vi "BCD to DEC.vi"(11 "BCD":u8) -> (3 "DEC":u16)   [LabVIEW 2014, in "LMH-Toolbox.lvlib"]
doc: "Convert a binary coded decimal to a decimal number."
uses:
  <vilib>/MakerHub/Toolbox/LMH-Toolbox.lvlib
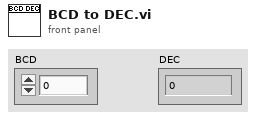
[diagram p1: front panel]
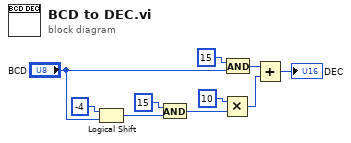
[diagram p0: block diagram]
diagram:
  n1 = Logical Shift(y=i16 -4, x="BCD") -> (x << y=w8:u8)
  n2 = And(x=u8 15, y=w8) -> (x .and. y?=w7:u8)
  n3 = Multiply(x=u16 10, y=w7) -> (x*y=w2:u16)
  n4 = And(x=u8 15, y="BCD") -> (x .and. y?=w3:u8)
  n5 = Add(x=w3, y=w2) -> (x+y=→"DEC":u16)
